vi "globalSetUp.vi"(8 "error in (no error)":errorcluster, 11 "testcase-CSMSyncMessage in":refnum<class "testcase-CSMMessage.lvclass">) -> (0 "error out":errorcluster, 3 "testcase-CSMSyncMessage out":refnum<class "testcase-CSMMessage.lvclass">)   [LabVIEW 2017, in "testcase-CSMMessage.lvclass"]
uses:
  testcase-CSMMessage.lvclass
  <vilib>/addons/_JKI Toolkits/VI Tester/TestCase.llb/TestCase.lvclass
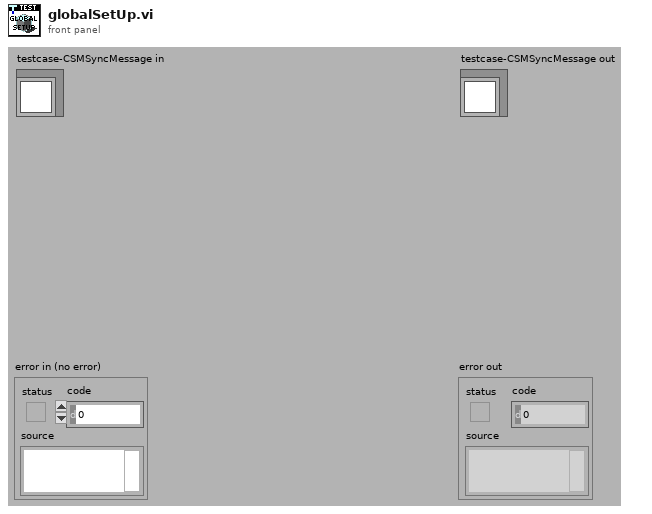
[diagram p1: front panel]
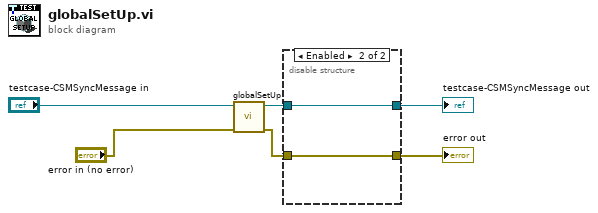
[diagram p0: block diagram]
diagram:
  n1 = call-parent "globalSetUp.vi"("error in (no error)"="error in (no error)", "TestCase in"="testcase-CSMSyncMessage in") -> ("error out"=w1:errorcluster, "TestCase out"=w3:refnum<class "testcase-CSMMessage.lvclass">)  [unwired: 8 in]
  n2 = disable-structure shown="Enabled" {
    disable-tunnel: w3 -> [w8 w10]
    disable-tunnel: [w8 w10] -> w6
    disable-tunnel: w1 -> [w7 w9]
    disable-tunnel: [w7 w9] -> w5
    frame Disabled {
    }
    frame Enabled {
    }
  }
  "error out" <- w5
  "testcase-CSMSyncMessage out" <- w6
